vi "Metadata FGV.vi"(9 "Sphere Indicator":T1=enum."Insulated Sphere", 10 "Control":enum16{"Get", "Set"}(ring), 11 "Metadata Fields In":T2) -> (3 "Metadata Fields Out":T2)   [LabVIEW 2013]
uses:
  Metadata Control.ctl
  avantesSpectrometer/Acquisition/Sphere Indicator.ctl
  avantesSpectrometer/AvaSpec.lvlib
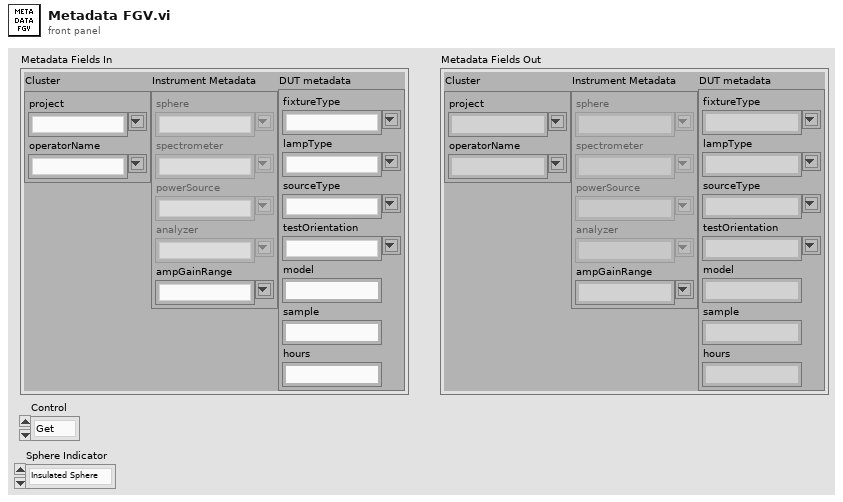
[diagram p1: front panel]
types:
  T1 = typedef "AvaSpec.lvlib/Sphere Indicator.ctl" = enum16{"Naked Sphere", "Insulated Sphere"}
  T2 = typedef "Metadata Control.ctl" = cluster{"Cluster":cluster{"project":string, "operatorName":string}, "Instrument Metadata":cluster{"sphere":string, "spectrometer":string, "powerSource":string, "analyzer":string, "ampGainRange":string}, "DUT metadata":cluster{"fixtureType":string, "lampType":string, "sourceType":string, "testOrientation":string, "model":string, "sample":string, "hours":string}}
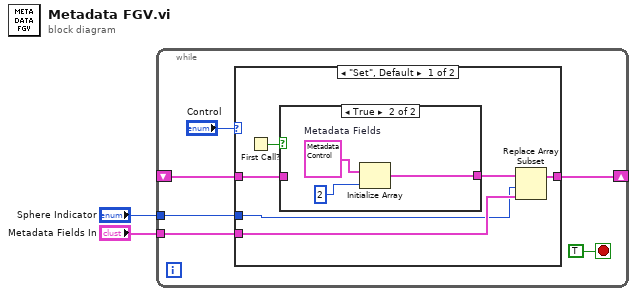
[diagram p0: block diagram]
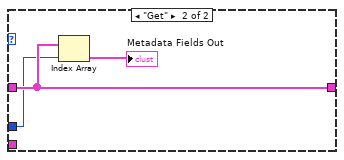
[diagram p3: hidden frame]
diagram:
  n1 = while {
    tunnel: "Metadata Fields In" -> [w7]
    shift-right: [w6] -> _
    shift-left: _ -> [w5]
    tunnel: "Sphere Indicator" -> [w3]
    stop <- TRUE stop-if-true
    n2 = case shown="\"Set\", Default" "Control" {
      tunnel: w7 -> [w10 _]
      tunnel: [w12 w21] -> w6
      tunnel: w5 -> [w11 w21]
      tunnel: w3 -> [w9 w20]
      frame "Set", Default {
        n3 = First Call?() -> (First Call?: T/F=w14:bool)
        n4 = case shown="True" w14 {
          tunnel: [w15 w16] -> w13
          tunnel: w11 -> [w15 _]
          frame False {
          }
          frame True {
            w18 = T2 {"Cluster"={"project"="", "operatorName"=""}, "Instrument Metadata"={"sphere"="NA", "spectrometer"="SMS 500", "powerSource"="Cal Inst 2253ix", "analyzer"="Yokogawa", "ampGainRange"=""}, "DUT metadata"={"fixtureType"="", "lampType"="", "sourceType"="", "testOrientation"="", "model"="", "sample"="", "hours"=""}}  # Metadata Fields
            n5 = Initialize Array(w18, 2 ("dimension size")) -> (w16:T2[])
          }
        }
        n6 = Replace Array Subset(array=w13, new element=w10, index=w9) -> (w12:T2[])
      }
      frame "Get" {
        n7 = Index Array(array=w21, index=w20) -> (element=→"Metadata Fields Out":T2)
      }
    }
  }
